vi "Boot Motor Controler.vi"(7 "Node ID":u8=1 min=1 max=127 step=1, 8 "error in (no error)":errorcluster, 11 "CANOpen Session in":refnum<k20>) -> (0 "error out":errorcluster, 1 "Success?":bool, 2 "Clustered SDO":T1, 3 "CANOpen Session out":refnum<k20>)   [LabVIEW 2016]
uses:
  Clustered SDO.ctl
  <vilib>/CANopenLib/CANOPEN.llb/CANopen SDO Create.vi
  Set into drive mode.vi
  Get Statusword.vi
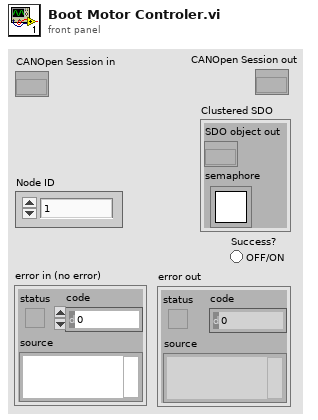
[diagram p1: front panel]
types:
  T1 = typedef "Clustered SDO.ctl" = cluster{"SDO object out":refnum<k20>, "semaphore":T2}
  T2 = typedef "Semaphore RefNum" = refnum<k1>
  T3 = typedef "Statusword.ctl" = cluster{"Ready to switch on":bool, "Switched on":bool, "Operation enabled":bool, "Fault":bool, "Voltage enabled":bool, "Quick stop":bool, "Switch on disabled":bool, "Warning":bool, "Remote":bool, "Target reached":bool, "Internal limit active":bool, "Operation mode specific":bool, "Manufacturer specific":bool}
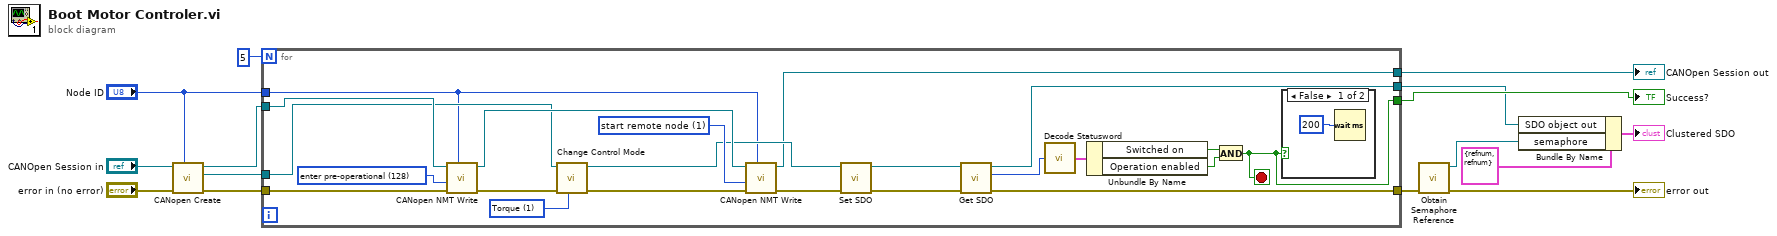
[diagram p0: block diagram]
diagram:
  n1 = call-poly <vilib>:"CANopen Create.vi"("node-ID"="Node ID", "error in (no error)"="error in (no error)", "interface object in"="CANOpen Session in") -> ("error out"=w8:errorcluster, "SDO object out"=w6:refnum<k20>, "interface object out"=w7:refnum<k20>)  [unwired: 6 in]
  n2 = for {
    N: 5 -> [_]
    tunnel: w8 -> [w24]
    tunnel: w7 -> [w23]
    tunnel: w6 -> [w22]
    tunnel: [w20] -> w5
    tunnel: [w19] -> w4
    tunnel: [w18] -> w3
    tunnel: [w17] -> w2
    tunnel: "Node ID" -> [w16]
    stop <- w18 stop-if-true
    w32 = u8 1 items=["Velocity"=2, "Torque"=1] ("Control Mode")
    w31 = u16 128 items=["start remote node"=1, "stop remote node"=2, "enter pre-operational"=128, "reset node"=129, "reset communication"=130] ("command")
    w33 = u16 1 items=["start remote node"=1, "stop remote node"=2, "enter pre-operational"=128, "reset node"=129, "reset communication"=130] ("command")
    n3 = call <vilib>:"CANopen NMT Write.vi"("node-ID (0)"=w16, "error in (no error)"=w24, "command"=w31, "interface object in"=w23) -> ("error out"=w30:errorcluster, "interface object out"=w28:refnum<k20>)  [unwired: 6 in]
    n4 = call "Change Control Mode.vi"("Control Mode"=w32, "error in (no error)"=w30, "SDO object in"=w22) -> ("error out"=w29:errorcluster, "SDO object out"=w21:refnum<k20>)  [unwired: 5 in, 2 out]
    n5 = call <vilib>:"CANopen NMT Write.vi"("node-ID (0)"=w16, "error in (no error)"=w29, "command"=w33, "interface object in"=w28) -> ("error out"=w34:errorcluster, "interface object out"=w20:refnum<k20>)  [unwired: 6 in]
    n6 = call-poly "Set SDO.vi"("error in (no error)"=w34, "SDO object in"=w21) -> ("error out"=w36:errorcluster, "SDO object out"=w37:refnum<k20>)  [unwired: 8 in]
    n7 = call-poly "Get SDO.vi"("error in (no error)"=w36, "SDO object in"=w37) -> ("error out"=w19:errorcluster, "Status word"=w35:u16, "SDO object out"=w17:refnum<k20>)  [unwired: 6 in, 1 out]
    n8 = call "Decode Statusword.vi"("Data"=w35) -> ("Status"=w27:T3)
    n9 = Unbundle By Name(w27) -> ("Switched on"=w25:bool, "Operation enabled"=w26:bool)
    n10 = And(x=w25, y=w26) -> (x .and. y?=w18:bool)
    n11 = case shown="False" w18 {
      frame False {
        n12 = Wait (ms)(milliseconds to wait=u32 200) -> ()  [unwired: 1 out]
      }
      frame True {
      }
    }
  }
  "CANOpen Session out" <- w5
  "Success?" <- w3
  n13 = call <vilib>:"Obtain Semaphore Reference.vi"("error in (no error)"=w4) -> ("error out"=→"error out":errorcluster, "semaphore"=w13:T2)  [unwired: 4 in, 1 out]
  n14 = Bundle By Name(cluster=T1 {"SDO object out"=refnum, "semaphore"=refnum} ("Clusterer SDO"), "SDO object out"=w2, "semaphore"=w13) -> (→"Clustered SDO":T1)
